vi "Unflatten Measurement Data and Store as Zip.vi"(8 "error in (no error)":errorcluster, 9 "Measurement Name":string, 10 "Measurement Data":string, 11 "Path to Store Measurement":path) -> (0 "error out":errorcluster, 3 "Folder Location":path)   [LabVIEW 2026, in "Client Controller.lvlib" / "Client Controller.lvclass"]
uses:
  Client Controller.lvclass
  <vilib>/zip/NI_Unzip.lvlib
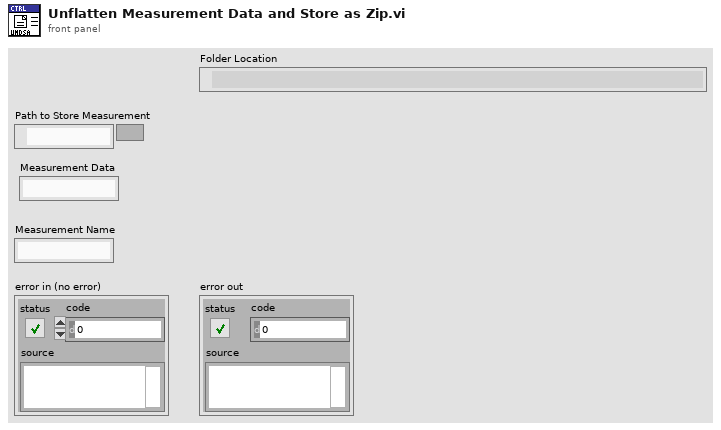
[diagram p1: front panel]
types:
  T1 = enum16{"big-endian, network order", "native, host order", "little-endian"}
  T2 = enum16{"open", "replace", "create", "open or create", "replace or create", "replace or create with confirmation"}
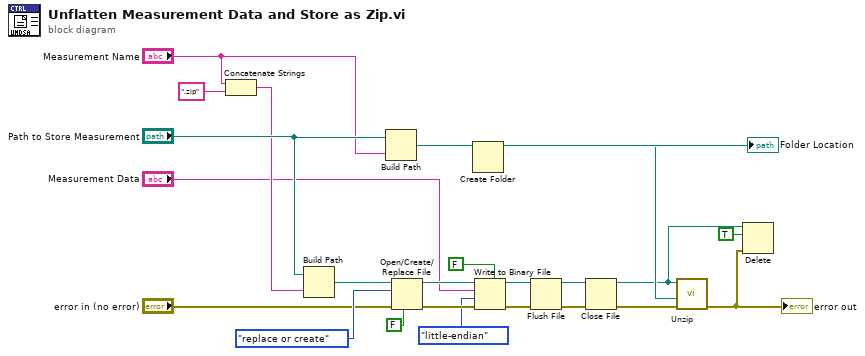
[diagram p0: block diagram]
diagram:
  n1 = Concatenate Strings("Measurement Name", ".zip" ("string")) -> (w6:string)
  n2 = Build Path(base path="Path to Store Measurement", name or relative path=w6) -> (appended path=w20:path)
  n3 = Build Path(base path="Path to Store Measurement", name or relative path="Measurement Name") -> (appended path=w14:path)
  "Folder Location" <- w14
  n4 = Open/Create/Replace File(file path (use dialog)=w20, error in="error in (no error)", operation (0:open)=T2."replace or create", disable buffering (F)=FALSE) -> (refnum out=w22:refnum<file>, error out=w21:errorcluster)  [unwired: 2 in, 1 out]
  n5 = Create Folder(path (use dialog)=w14) -> (created path=w13:path)  [unwired: 2 in, 2 out]
  n6 = Write to Binary File(file (use dialog)=w22, data="Measurement Data", error in=w21, 5:FALSE ("prepend array or string size? (T)"), 9:T1."little-endian" ("byte order (0:big-endian, network order)")) -> (refnum out=w16:refnum<file>, error out=w12:errorcluster)  [unwired: 1 in, 1 out]
  n7 = Flush File(refnum=w16, error in=w12) -> (refnum out=w15:refnum<file>, error out=w11:errorcluster)
  n8 = Close File(refnum=w15, error in=w11) -> (path=w4:path, error out=w10:errorcluster)
  n9 = call <vilib>:"Unzip.vi"("error in (no error)"=w10, "Target directory (same as Zip file if empty)"=w13, "Zip file"=w4) -> ("error out"=w5:errorcluster)  [unwired: 6 in, 2 out]
  "error out" <- w5
  n10 = Delete(path (use dialog)=w4, entire hierarchy (F)=TRUE, error in=w5) -> ()  [unwired: 2 in, 3 out]
